vi "SMU_Set Current Level and Range.vi"(5 "current level":dbl=1e-05 format="%#_13p", 7 "current range":dbl format="%#_6p", 8 "error in (no error)":errorcluster, 10 "Pins":string[](array[string])=["RF1", "RF2", "RF3", "RF4"], 11 "Semiconductor Module Context":T1) -> (0 "error out":errorcluster, 3 "Semiconductor Module Context Out":T1)   [LabVIEW 2013]
uses:
  <vilib>/NI_TestStand_SemiconductorModule/NI_TestStand_Semiconductor_Module.lvlibp/PinMap/General/SemiconductorModuleContext.ctl
  <vilib>/NI_TestStand_SemiconductorModule/NI_TestStand_Semiconductor_Module.lvlibp/PinMap/DC Power/PinsToNIDCPowerSessions.vi
  <vilib>/NI_TestStand_SemiconductorModule/NI_TestStand_Semiconductor_Module.lvlibp
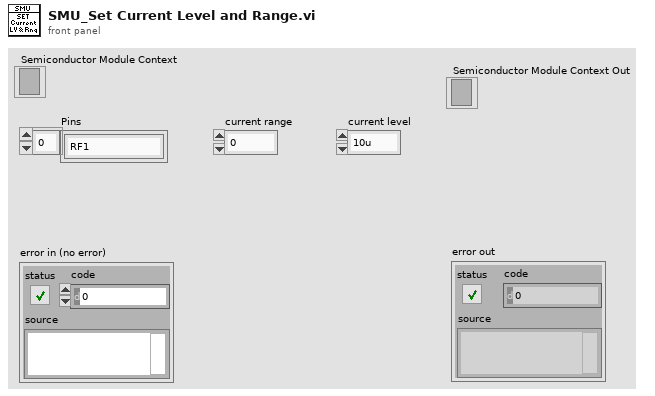
[diagram p1: front panel]
types:
  T1 = typedef "NI_TestStand_Semiconductor_Module.lvlibp/SemiconductorModuleContext.ctl" = refnum<k7>
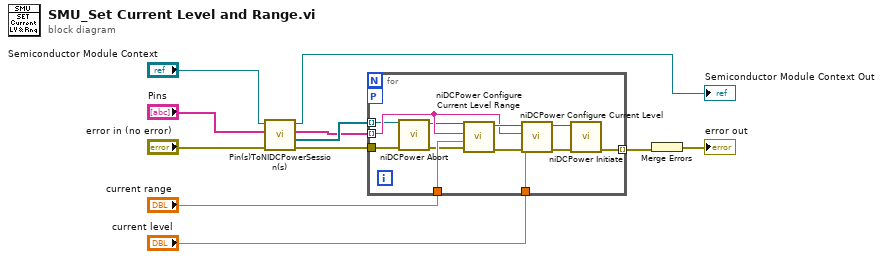
[diagram p0: block diagram]
diagram:
  n1 = call-poly <vilib>:"Pin(s)ToNIDCPowerSession(s).vi"("error in (no error)"="error in (no error)", "Pins"="Pins", "Semiconductor Module Context"="Semiconductor Module Context") -> ("error out"=w11:errorcluster, "Instrument Sessions"=w10:refnum<k15>[], "Channel Lists"=w9:string[], "Semiconductor Module Context Out"=→"Semiconductor Module Context Out":T1)  [unwired: 4 in, 1 out]
  n2 = for {
    tunnel: w11 -> [w17]
    tunnel: w10 -> [w18] mode=indexing
    tunnel: w9 -> [w21] mode=indexing
    workers-P: _ -> [_]
    tunnel: [w13] -> w3 mode=indexing
    tunnel: "current range" -> [w20]
    tunnel: "current level" -> [w19]
    n3 = call <instrlib>:"niDCPower Abort.vi"("error in (no error)"=w17, "instrument handle"=w18) -> ("error out"=w16:errorcluster, "instrument handle out"=w15:refnum<k15>)  [unwired: 8 in]
    n4 = call <instrlib>:"niDCPower Configure Current Level Range.vi"("error in (no error)"=w16, "current level range"=w20, "channel name"=w21, "instrument handle"=w15) -> ("error out"=w23:errorcluster, "instrument handle out"=w22:refnum<k15>)  [unwired: 6 in]
    n5 = call <instrlib>:"niDCPower Configure Current Level.vi"("error in (no error)"=w23, "current level"=w19, "channel name"=w21, "instrument handle"=w22) -> ("error out"=w14:errorcluster, "instrument handle out"=w12:refnum<k15>)  [unwired: 6 in]
    n6 = call <instrlib>:"niDCPower Initiate.vi"("error in (no error)"=w14, "instrument handle"=w12) -> ("error out"=w13:errorcluster)  [unwired: 8 in, 1 out]
  }
  n7 = Merge Errors(w3) -> (→"error out":errorcluster)
